vi "Cache Power Meter.vi"(0 "Power Meter Base in":refnum<class "Power Meter Base.lvclass">, 11 "error in (no error)":errorcluster) -> (4 "Power Meter Base out":refnum<class "Power Meter Base.lvclass">, 15 "error out":errorcluster)   [LabVIEW 2023, in "RFFixtureCharact.Instruments.lvlib" / "Power Meter Factory.lvclass"]
uses:
  Power Meter Factory.lvclass
  Power Meter Base/Power Meter Base.lvclass
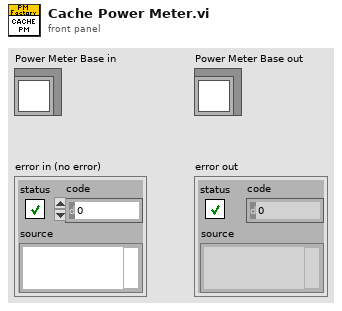
[diagram p1: front panel]
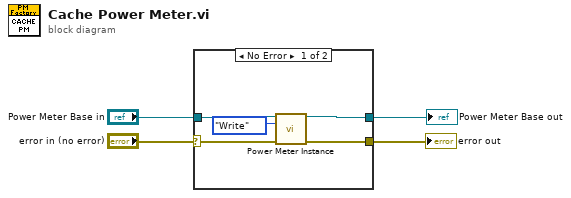
[diagram p0: block diagram]
diagram:
  n1 = case shown="No Error" "error in (no error)" {
    selector: "error in (no error)" -> [w9 w11]
    tunnel: [w8 w11] -> w3
    tunnel: "Power Meter Base in" -> [w7 w10]
    tunnel: [w6 w10] -> w1
    frame No Error {
      n2 = call "Power Meter Instance.vi"("Power Meter in"=w7, "Operation"=enum16{"Read", "Write", "Clear"}."Write", "error in (no error)"=w9) -> ("Power Meter out"=w6:refnum<class "Power Meter Base.lvclass">, "error out"=w8:errorcluster)  [unwired: 10 in, 1 out]
    }
    frame Error {
    }
  }
  "error out" <- w3
  "Power Meter Base out" <- w1
